vi "exp_1_excersises.vi"() -> ()   [LabVIEW 2026]
panel:
  in  "Numeric":csg
  out "r * e^(i*theta)":cdb
  out "theta":dbl
  out "r":dbl
  in  "Basic":dbl
  out "TAKE-HOME SALARY":dbl
  out "Y":bool
  in  "D":bool
  in  "C":bool
  in  "B":bool
  in  "A":bool
  out "output variable":dbl
  out "y":dbl
  in  "b":dbl
  in  "a":dbl
  out "METER":dbl
  in  "INCHES":dbl
  # "1. Write a program to convert inches to meters"
  # "2. Write a program to perform y=4.5a*logb+10(a+b)\n using functions and formula node."
  # "a) using functions"
  # "b) using node"
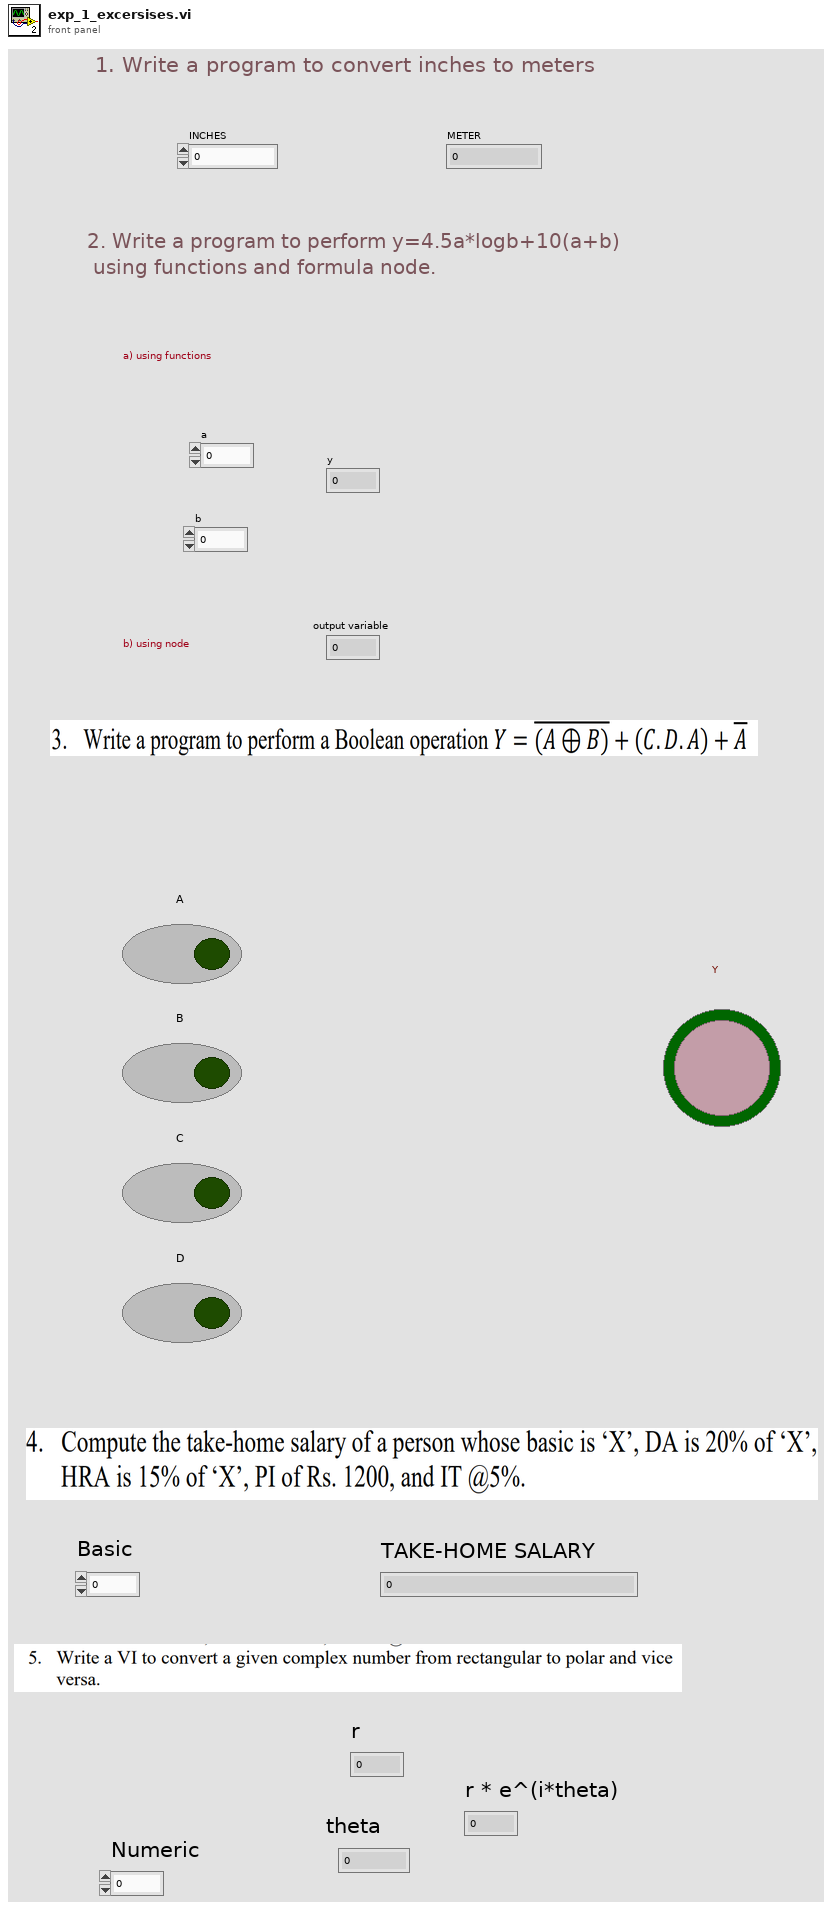
[diagram p1: front panel]
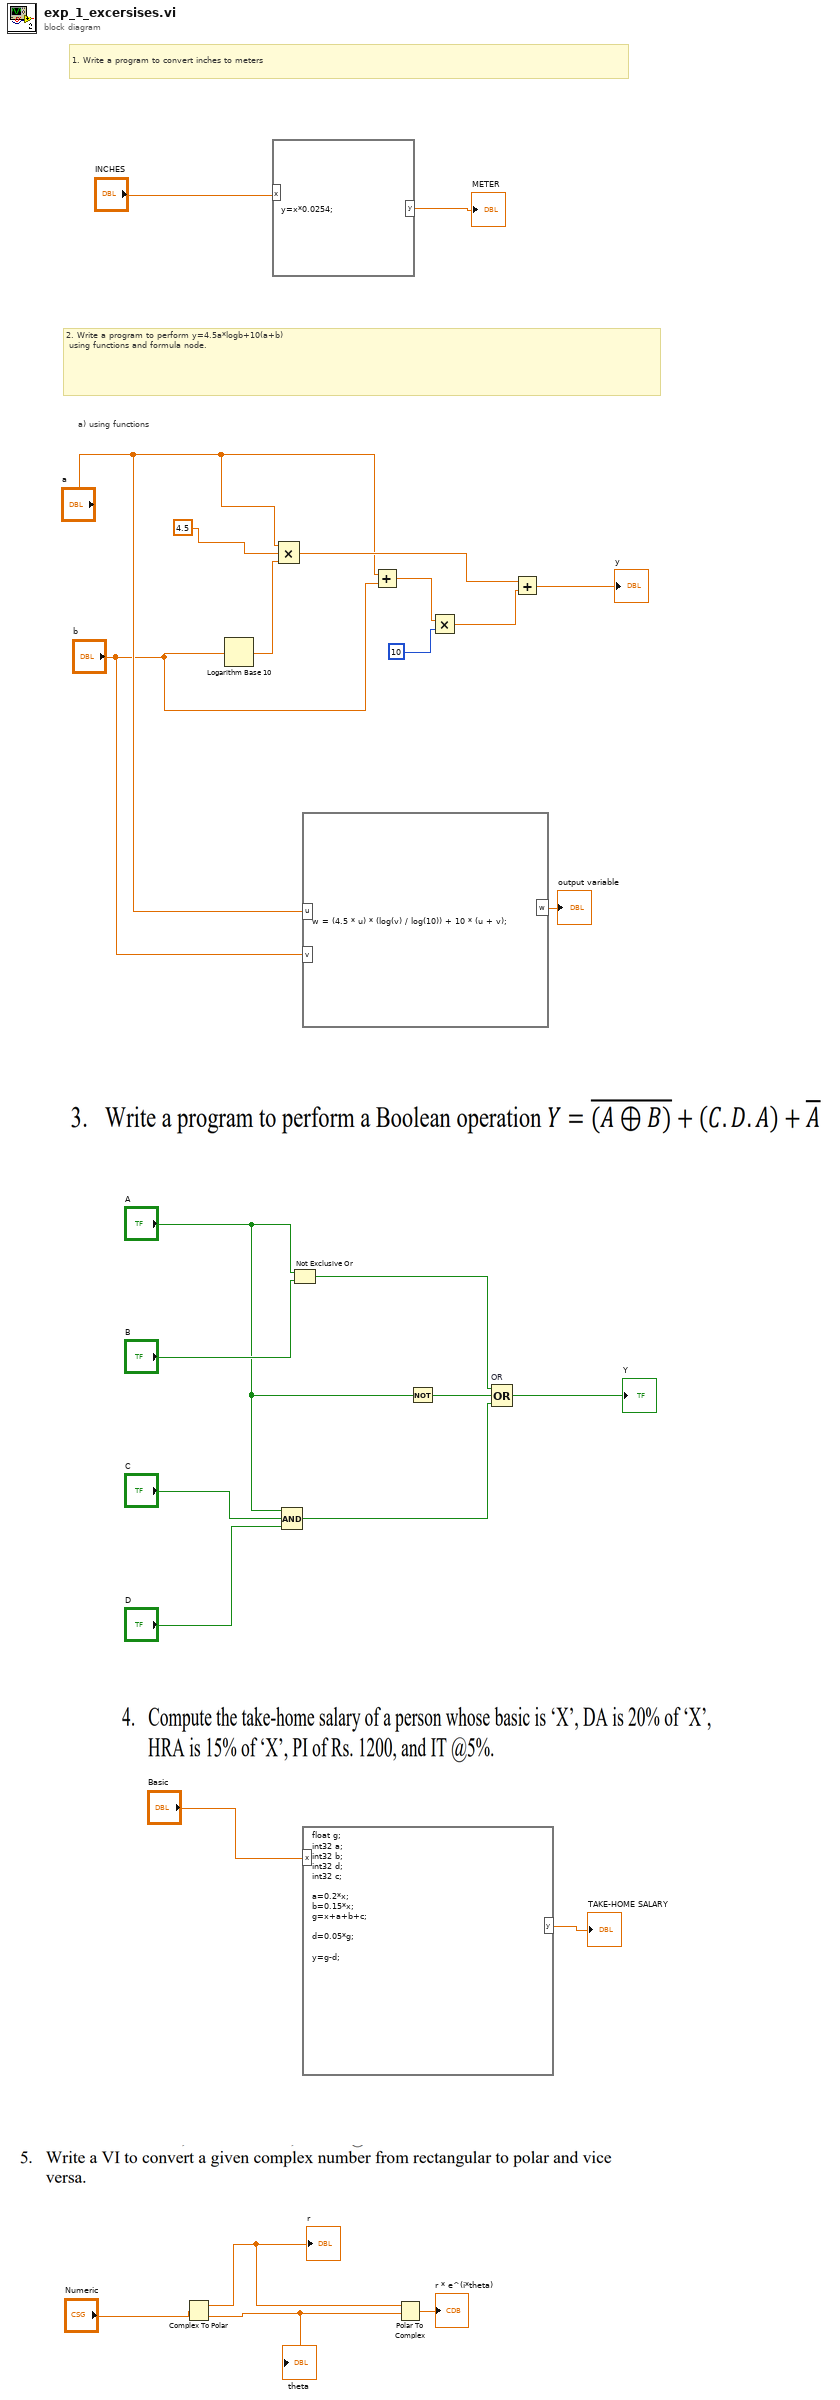
[diagram p0: block diagram]
diagram:
  # "2. Write a program to perform y=4.5a*logb+10(a+b)\n using functions and formula node."
  # "a) using functions"
  # "1. Write a program to convert inches to meters"
  n1 = Complex To Polar(r * e^(i*theta)="Numeric") -> (r=w3:sgl, theta=w2:sgl)
  "r" <- w3
  "theta" <- w2
  n2 = Logarithm Base 10(1:"b") -> (0:w23:dbl)
  n3 = formula code="y=x*0.0254;"("x"="INCHES") -> ("y"=→"METER":dbl)
  n4 = Compound Arithmetic op=MULTIPLY("a", 4.5, w23) -> (w20:dbl)
  n5 = Compound Arithmetic op=AND("A", "C", "D") -> (w8:bool)
  n6 = Not Exclusive Or(1:"B", 2:"A") -> (0:w13:bool)
  n7 = formula code="w = (4.5 * u) * (log(v) / log(10)) + 10 * (u + v);"("u"="a", "v"="b") -> ("w"=→"output variable":dbl)
  n8 = formula code="float g;\nint32 a;\nint32 b;\nint32 d;\nint32 c;\n\na=0.2*x;\nb=0.15*x;\ng=x+a+b+c;\n\nd=0.05*g;\n\ny=g-d;"("x"="Basic") -> ("y"=→"TAKE-HOME SALARY":dbl)
  n9 = Add(x="a", y="b") -> (x+y=w22:dbl)
  n10 = Polar To Complex(1:w2, 2:w3) -> (0:→"r * e^(i*theta)":csg)
  n11 = Not(x="A") -> (.not. x?=w10:bool)
  n12 = Multiply(x=w22, y=10) -> (x*y=w19:dbl)
  n13 = Compound Arithmetic op=OR "OR"(w13, w10, w8) -> (→"Y":bool)
  n14 = Add(x=w20, y=w19) -> (x+y=→"y":dbl)
